vi "Send.vi"(7 "High Priority (F)":bool, 8 "error in (no error)":errorcluster, 9 "Data":variant, 10 "ID":string, 11 "MessageQ in":refnum<class "MessageQ.lvclass">) -> (0 "error out":errorcluster, 3 "MessageQ out":refnum<class "MessageQ.lvclass">)   [LabVIEW 2020, in "Volatus.lvlib" / "MessageQ.lvclass"]
uses:
  MessageQ.lvclass
  MessageQ.lvclass/MessageQ.ctl
  Message.ctl
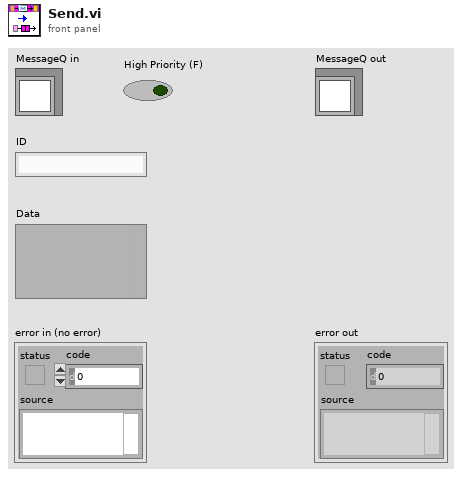
[diagram p1: front panel]
types:
  T1 = typedef "Volatus.lvlib/MessageQ.lvclass/Message.ctl" = cluster{"ID":string, "Data":variant}
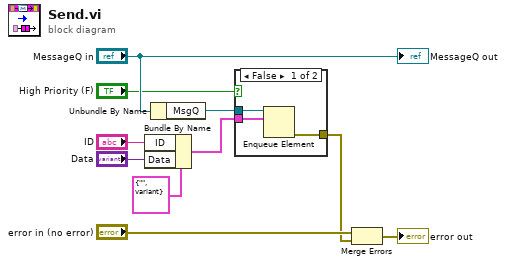
[diagram p0: block diagram]
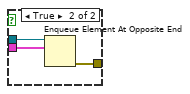
[diagram p2: hidden frame]
diagram:
  n1 = Bundle By Name(cluster=T1 {"ID"="", "Data"=variant} ("Message"), "ID"="ID", "Data"="Data") -> (w4:T1)
  n2 = Unbundle By Name("MessageQ in") -> ("MsgQ"=w8:refnum<queue>)
  n3 = case shown="False" "High Priority (F)" {
    tunnel: w8 -> [w13 w16]
    tunnel: w4 -> [w12 w15]
    tunnel: [w11 w14] -> w1
    frame False {
      n4 = Enqueue Element(queue=w13, element=w12) -> (error out=w11:errorcluster)  [unwired: 2 in, 2 out]
    }
    frame True {
      n5 = Enqueue Element At Opposite End(queue=w16, element=w15) -> (error out=w14:errorcluster)  [unwired: 2 in, 2 out]
    }
  }
  n6 = Merge Errors("error in (no error)", w1) -> (→"error out":errorcluster)
  "MessageQ out" <- "MessageQ in"
